vi "Conversie C2.vi"(0 "Array":string[](array[string])) -> (1 "12 bit LSB value (x)":i32, 2 "12 bit LSB value (y)":i32, 3 "12 bit LSB value (z)":i32, 4 "12 bit Field value (mT) X":dbl, 6 "12 bit Field value (mT) Y":dbl, 8 "12 bit Field value (mT) Z":dbl, 10 "12 bit temp (C)":dbl, 14 "12 bit LSB value (temp)":i32, 15 "FRM":i32)   [LabVIEW 2020]
panel:
  in  "Tab Control":enum32{"Page 1", "Page 2"}(tab)
  out "8 bit MSB value Z":i32
  out "8 bit Field value (mT) Z":dbl
  out "8 bit MSB value X":i32
  out "8 bit Field value (mT) X":dbl
  out "8 bit MSB value Y":i32
  out "8 bit Field value (mT) Y":dbl
  out "CH":i32
  out "T":i32
  out "FF":i32
  out "PD":i32
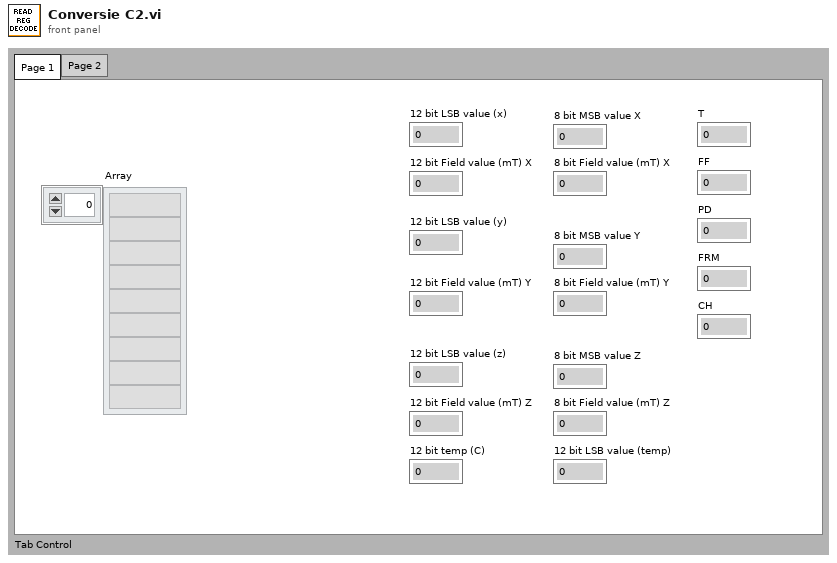
[diagram p1: front panel]
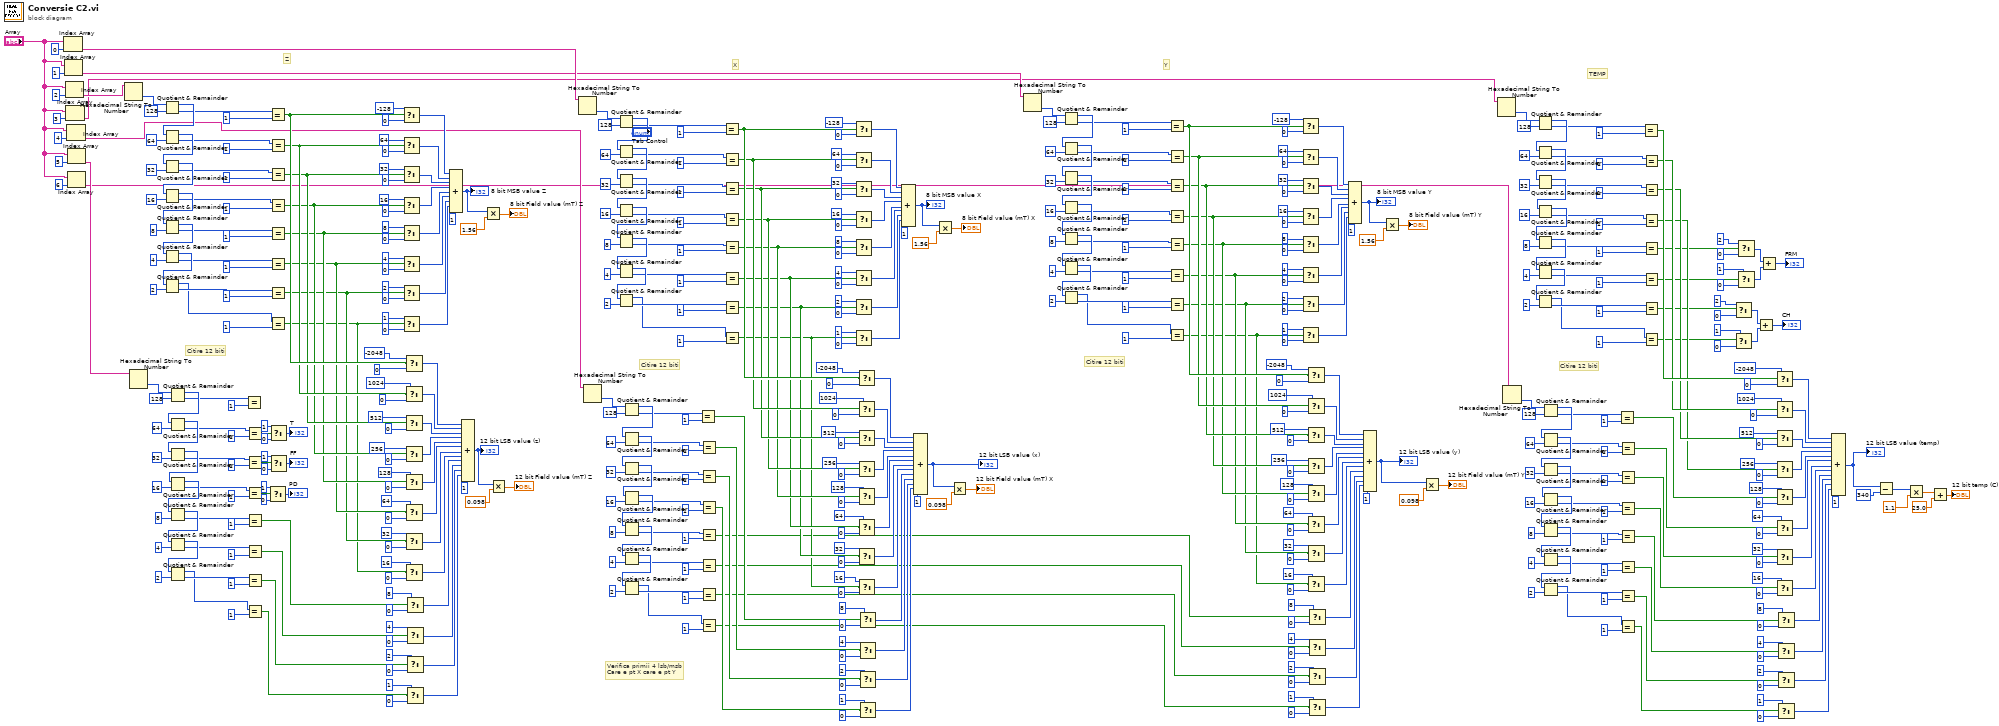
[diagram p0: block diagram]
diagram:
  # "Verifica primii 4 lsb/msb\nCare e pt X care e pt Y"
  # "TEMP"
  # "Y"
  # "X"
  # "Z"
  # "Citire 12 biti"
  # "Citire 12 biti"
  # "Citire 12 biti"
  # "Citire 12 biti"
  n1 = Index Array(array="Array", index=0) -> (element=w22:string)
  n2 = Index Array(array="Array", index=1) -> (element=w16:string)
  n3 = Index Array(array="Array", index=2) -> (element=w15:string)
  n4 = Index Array(array="Array", index=3) -> (element=w14:string)
  n5 = Index Array(array="Array", index=4) -> (element=w13:string)
  n6 = Index Array(array="Array", index=5) -> (element=w12:string)
  n7 = Index Array(array="Array", index=6) -> (element=w9:string)
  n8 = Hexadecimal String To Number(string=w15) -> (number=w522:u32)  [unwired: 2 in, 1 out]
  n9 = Hexadecimal String To Number(string=w12) -> (number=w466:u32)  [unwired: 2 in, 1 out]
  n10 = Quotient & Remainder(x=w522, y=u8 128) -> (x-y*floor(x/y)=w542:u32, floor(x/y)=w530:u32)
  n11 = Quotient & Remainder(x=w542, y=u8 64) -> (x-y*floor(x/y)=w541:u32, floor(x/y)=w524:u32)
  n12 = Quotient & Remainder(x=w541, y=u8 32) -> (x-y*floor(x/y)=w540:u32, floor(x/y)=w529:u32)
  n13 = Quotient & Remainder(x=w540, y=u8 16) -> (x-y*floor(x/y)=w539:u32, floor(x/y)=w528:u32)
  n14 = Quotient & Remainder(x=w539, y=u8 8) -> (x-y*floor(x/y)=w538:u32, floor(x/y)=w527:u32)
  n15 = Quotient & Remainder(x=w538, y=u8 4) -> (x-y*floor(x/y)=w537:u32, floor(x/y)=w526:u32)
  n16 = Quotient & Remainder(x=w537, y=u8 2) -> (x-y*floor(x/y)=w523:u32, floor(x/y)=w525:u32)
  n17 = Quotient & Remainder(x=w466, y=u8 128) -> (x-y*floor(x/y)=w486:u32, floor(x/y)=w474:u32)
  n18 = Quotient & Remainder(x=w486, y=u8 64) -> (x-y*floor(x/y)=w485:u32, floor(x/y)=w468:u32)
  n19 = Quotient & Remainder(x=w485, y=u8 32) -> (x-y*floor(x/y)=w484:u32, floor(x/y)=w473:u32)
  n20 = Quotient & Remainder(x=w484, y=u8 16) -> (x-y*floor(x/y)=w483:u32, floor(x/y)=w472:u32)
  n21 = Quotient & Remainder(x=w483, y=u8 8) -> (x-y*floor(x/y)=w482:u32, floor(x/y)=w471:u32)
  n22 = Quotient & Remainder(x=w482, y=u8 4) -> (x-y*floor(x/y)=w481:u32, floor(x/y)=w470:u32)
  n23 = Quotient & Remainder(x=w481, y=u8 2) -> (x-y*floor(x/y)=w467:u32, floor(x/y)=w469:u32)
  n24 = Equal?(x=w474, y=u8 1) -> ()  [unwired: 1 out]
  n25 = Equal?(x=w468, y=u8 1) -> (x = y?=w33:bool)
  n26 = Equal?(x=w473, y=u8 1) -> (x = y?=w28:bool)
  n27 = Equal?(x=w472, y=u8 1) -> (x = y?=w24:bool)
  n28 = Equal?(x=w471, y=u8 1) -> (x = y?=w156:bool)
  n29 = Equal?(x=w470, y=u8 1) -> (x = y?=w155:bool)
  n30 = Equal?(x=w469, y=u8 1) -> (x = y?=w154:bool)
  n31 = Equal?(x=w467, y=u8 1) -> (x = y?=w153:bool)
  n32 = Equal?(x=w530, y=u8 1) -> (x = y?=w164:bool)
  n33 = Select(t=u8 1 ("f"), s=w24, f=u8 0 ("t")) -> (s? t:f=→"PD":u8)
  n34 = Equal?(x=w524, y=u8 1) -> (x = y?=w163:bool)
  n35 = Equal?(x=w529, y=u8 1) -> (x = y?=w162:bool)
  n36 = Equal?(x=w528, y=u8 1) -> (x = y?=w161:bool)
  n37 = Equal?(x=w527, y=u8 1) -> (x = y?=w160:bool)
  n38 = Equal?(x=w526, y=u8 1) -> (x = y?=w159:bool)
  n39 = Equal?(x=w525, y=u8 1) -> (x = y?=w158:bool)
  n40 = Equal?(x=w523, y=u8 1) -> (x = y?=w157:bool)
  n41 = Select(t=u8 1 ("f"), s=w33, f=u8 0 ("t")) -> (s? t:f=→"T":u8)
  n42 = Select(t=u8 1 ("f"), s=w28, f=u8 0 ("t")) -> (s? t:f=→"FF":u8)
  n43 = Select(t=-128, s=w164, f=u8 0 ("t")) -> (s? t:f=w507:i32)
  n44 = Select(t=u8 64, s=w163, f=u8 0) -> (s? t:f=w506:u8)
  n45 = Select(t=u8 32, s=w162, f=u8 0) -> (s? t:f=w505:u8)
  n46 = Select(t=u8 16, s=w161, f=u8 0) -> (s? t:f=w504:u8)
  n47 = Select(t=u8 8, s=w160, f=u8 0) -> (s? t:f=w503:u8)
  n48 = Select(t=u8 4, s=w159, f=u8 0) -> (s? t:f=w502:u8)
  n49 = Select(t=u8 2, s=w158, f=u8 0) -> (s? t:f=w501:u8)
  n50 = Select(t=u8 1, s=w157, f=u8 0) -> (s? t:f=w500:u8)
  n51 = Select(t=-2048, s=w164, f=u8 0 ("t")) -> (s? t:f=w201:i32)
  n52 = Select(t=1024, s=w163, f=u8 0 ("t")) -> (s? t:f=w200:i32)
  n53 = Select(t=512, s=w162, f=u8 0 ("t")) -> (s? t:f=w199:i32)
  n54 = Select(t=256, s=w161, f=u8 0 ("t")) -> (s? t:f=w198:i32)
  n55 = Select(t=u8 128 ("f"), s=w160, f=u8 0 ("t")) -> (s? t:f=w197:u8)
  n56 = Select(t=u8 64 ("f"), s=w159, f=u8 0 ("t")) -> (s? t:f=w196:u8)
  n57 = Select(t=u8 32 ("f"), s=w158, f=u8 0 ("t")) -> (s? t:f=w195:u8)
  n58 = Select(t=u8 16 ("f"), s=w157, f=u8 0 ("t")) -> (s? t:f=w194:u8)
  n59 = Select(t=u8 8 ("f"), s=w156, f=u8 0 ("t")) -> (s? t:f=w192:u8)
  n60 = Select(t=u8 4 ("f"), s=w155, f=u8 0 ("t")) -> (s? t:f=w191:u8)
  n61 = Select(t=u8 2 ("f"), s=w154, f=u8 0 ("t")) -> (s? t:f=w190:u8)
  n62 = Select(t=u8 1 ("f"), s=w153, f=u8 0 ("t")) -> (s? t:f=w189:u8)
  n63 = Compound Arithmetic op=ADD(w507, w506, w505, w504, w503, w502, w501, w500, u8 1 ("Input")) -> (w498:i32)
  "8 bit MSB value Z" <- w498
  n64 = Compound Arithmetic op=ADD(w201, w200, w199, w198, w197, w196, w195, w194, w192, w191, w190, w189, u8 1 ("Input")) -> (w152:i32)
  "12 bit LSB value (z)" <- w152
  n65 = Multiply(x=w498, y=1.56) -> (x*y=→"8 bit Field value (mT) Z":dbl)
  n66 = Multiply(x=w152, y=0.098) -> (x*y=→"12 bit Field value (mT) Z":dbl)
  n67 = Hexadecimal String To Number(string=w22) -> (number=w434:u32)  [unwired: 2 in, 1 out]
  n68 = Hexadecimal String To Number(string=w13) -> (number=w378:u32)  [unwired: 2 in, 1 out]
  n69 = Quotient & Remainder(x=w434, y=u8 128) -> (x-y*floor(x/y)=w454:u32, floor(x/y)=w442:u32)
  n70 = Quotient & Remainder(x=w454, y=u8 64) -> (x-y*floor(x/y)=w453:u32, floor(x/y)=w436:u32)
  n71 = Quotient & Remainder(x=w453, y=u8 32) -> (x-y*floor(x/y)=w452:u32, floor(x/y)=w441:u32)
  n72 = Quotient & Remainder(x=w452, y=u8 16) -> (x-y*floor(x/y)=w451:u32, floor(x/y)=w440:u32)
  n73 = Quotient & Remainder(x=w451, y=u8 8) -> (x-y*floor(x/y)=w450:u32, floor(x/y)=w439:u32)
  n74 = Quotient & Remainder(x=w450, y=u8 4) -> (x-y*floor(x/y)=w449:u32, floor(x/y)=w438:u32)
  n75 = Quotient & Remainder(x=w449, y=u8 2) -> (x-y*floor(x/y)=w435:u32, floor(x/y)=w437:u32)
  n76 = Quotient & Remainder(x=w378, y=u8 128) -> (x-y*floor(x/y)=w398:u32, floor(x/y)=w386:u32)
  n77 = Quotient & Remainder(x=w398, y=u8 64) -> (x-y*floor(x/y)=w397:u32, floor(x/y)=w380:u32)
  n78 = Quotient & Remainder(x=w397, y=u8 32) -> (x-y*floor(x/y)=w396:u32, floor(x/y)=w385:u32)
  n79 = Quotient & Remainder(x=w396, y=u8 16) -> (x-y*floor(x/y)=w395:u32, floor(x/y)=w384:u32)
  n80 = Quotient & Remainder(x=w395, y=u8 8) -> (x-y*floor(x/y)=w394:u32, floor(x/y)=w383:u32)
  n81 = Quotient & Remainder(x=w394, y=u8 4) -> (x-y*floor(x/y)=w393:u32, floor(x/y)=w382:u32)
  n82 = Quotient & Remainder(x=w393, y=u8 2) -> (x-y*floor(x/y)=w379:u32, floor(x/y)=w381:u32)
  n83 = Equal?(x=w386, y=u8 1) -> (x = y?=w8:bool)
  n84 = Equal?(x=w380, y=u8 1) -> (x = y?=w7:bool)
  n85 = Equal?(x=w385, y=u8 1) -> (x = y?=w6:bool)
  n86 = Equal?(x=w384, y=u8 1) -> (x = y?=w5:bool)
  n87 = Equal?(x=w383, y=u8 1) -> (x = y?=w4:bool)
  n88 = Equal?(x=w382, y=u8 1) -> (x = y?=w3:bool)
  n89 = Equal?(x=w381, y=u8 1) -> (x = y?=w2:bool)
  n90 = Equal?(x=w379, y=u8 1) -> (x = y?=w1:bool)
  n91 = Equal?(x=w442, y=u8 1) -> (x = y?=w115:bool)
  n92 = Equal?(x=w436, y=u8 1) -> (x = y?=w114:bool)
  n93 = Equal?(x=w441, y=u8 1) -> (x = y?=w113:bool)
  n94 = Equal?(x=w440, y=u8 1) -> (x = y?=w112:bool)
  n95 = Equal?(x=w439, y=u8 1) -> (x = y?=w111:bool)
  n96 = Equal?(x=w438, y=u8 1) -> (x = y?=w110:bool)
  n97 = Equal?(x=w437, y=u8 1) -> (x = y?=w109:bool)
  n98 = Equal?(x=w435, y=u8 1) -> (x = y?=w108:bool)
  n99 = Select(t=-128, s=w115, f=u8 0 ("t")) -> (s? t:f=w419:i32)
  n100 = Select(t=u8 64, s=w114, f=u8 0) -> (s? t:f=w418:u8)
  n101 = Select(t=u8 32, s=w113, f=u8 0) -> (s? t:f=w417:u8)
  n102 = Select(t=u8 16, s=w112, f=u8 0) -> (s? t:f=w416:u8)
  n103 = Select(t=u8 8, s=w111, f=u8 0) -> (s? t:f=w415:u8)
  n104 = Select(t=u8 4, s=w110, f=u8 0) -> (s? t:f=w414:u8)
  n105 = Select(t=u8 2, s=w109, f=u8 0) -> (s? t:f=w413:u8)
  n106 = Select(t=u8 1, s=w108, f=u8 0) -> (s? t:f=w412:u8)
  n107 = Select(t=-2048, s=w115, f=u8 0 ("t")) -> (s? t:f=w151:i32)
  n108 = Select(t=1024, s=w114, f=u8 0 ("t")) -> (s? t:f=w150:i32)
  n109 = Select(t=512, s=w113, f=u8 0 ("t")) -> (s? t:f=w149:i32)
  n110 = Select(t=256, s=w112, f=u8 0 ("t")) -> (s? t:f=w148:i32)
  n111 = Select(t=u8 128 ("f"), s=w111, f=u8 0 ("t")) -> (s? t:f=w147:u8)
  n112 = Select(t=u8 64 ("f"), s=w110, f=u8 0 ("t")) -> (s? t:f=w146:u8)
  n113 = Select(t=u8 32 ("f"), s=w109, f=u8 0 ("t")) -> (s? t:f=w145:u8)
  n114 = Select(t=u8 16 ("f"), s=w108, f=u8 0 ("t")) -> (s? t:f=w144:u8)
  n115 = Select(t=u8 8 ("f"), s=w8, f=u8 0 ("t")) -> (s? t:f=w142:u8)
  n116 = Select(t=u8 4 ("f"), s=w7, f=u8 0 ("t")) -> (s? t:f=w141:u8)
  n117 = Select(t=u8 2 ("f"), s=w6, f=u8 0 ("t")) -> (s? t:f=w140:u8)
  n118 = Select(t=u8 1 ("f"), s=w5, f=u8 0 ("t")) -> (s? t:f=w139:u8)
  n119 = Compound Arithmetic op=ADD(w419, w418, w417, w416, w415, w414, w413, w412, u8 1 ("Input")) -> (w410:i32)
  "8 bit MSB value X" <- w410
  n120 = Compound Arithmetic op=ADD(w151, w150, w149, w148, w147, w146, w145, w144, w142, w141, w140, w139, u8 1 ("Input")) -> (w107:i32)
  "12 bit LSB value (x)" <- w107
  n121 = Multiply(x=w410, y=1.56) -> (x*y=→"8 bit Field value (mT) X":dbl)
  n122 = Multiply(x=w107, y=0.098) -> (x*y=→"12 bit Field value (mT) X":dbl)
  n123 = Hexadecimal String To Number(string=w16) -> (number=w346:u32)  [unwired: 2 in, 1 out]
  n124 = Quotient & Remainder(x=w346, y=u8 128) -> (x-y*floor(x/y)=w366:u32, floor(x/y)=w354:u32)
  n125 = Quotient & Remainder(x=w366, y=u8 64) -> (x-y*floor(x/y)=w365:u32, floor(x/y)=w348:u32)
  n126 = Quotient & Remainder(x=w365, y=u8 32) -> (x-y*floor(x/y)=w364:u32, floor(x/y)=w353:u32)
  n127 = Quotient & Remainder(x=w364, y=u8 16) -> (x-y*floor(x/y)=w363:u32, floor(x/y)=w352:u32)
  n128 = Quotient & Remainder(x=w363, y=u8 8) -> (x-y*floor(x/y)=w362:u32, floor(x/y)=w351:u32)
  n129 = Quotient & Remainder(x=w362, y=u8 4) -> (x-y*floor(x/y)=w361:u32, floor(x/y)=w350:u32)
  n130 = Quotient & Remainder(x=w361, y=u8 2) -> (x-y*floor(x/y)=w347:u32, floor(x/y)=w349:u32)
  n131 = Equal?(x=w354, y=u8 1) -> (x = y?=w70:bool)
  n132 = Equal?(x=w348, y=u8 1) -> (x = y?=w69:bool)
  n133 = Equal?(x=w353, y=u8 1) -> (x = y?=w68:bool)
  n134 = Equal?(x=w352, y=u8 1) -> (x = y?=w67:bool)
  n135 = Equal?(x=w351, y=u8 1) -> (x = y?=w66:bool)
  n136 = Equal?(x=w350, y=u8 1) -> (x = y?=w65:bool)
  n137 = Equal?(x=w349, y=u8 1) -> (x = y?=w64:bool)
  n138 = Equal?(x=w347, y=u8 1) -> (x = y?=w63:bool)
  n139 = Select(t=-128, s=w70, f=u8 0 ("t")) -> (s? t:f=w331:i32)
  n140 = Select(t=u8 64, s=w69, f=u8 0) -> (s? t:f=w330:u8)
  n141 = Select(t=u8 32, s=w68, f=u8 0) -> (s? t:f=w329:u8)
  n142 = Select(t=u8 16, s=w67, f=u8 0) -> (s? t:f=w328:u8)
  n143 = Select(t=u8 8, s=w66, f=u8 0) -> (s? t:f=w327:u8)
  n144 = Select(t=u8 4, s=w65, f=u8 0) -> (s? t:f=w326:u8)
  n145 = Select(t=u8 2, s=w64, f=u8 0) -> (s? t:f=w325:u8)
  n146 = Select(t=u8 1, s=w63, f=u8 0) -> (s? t:f=w324:u8)
  n147 = Select(t=-2048, s=w70, f=u8 0 ("t")) -> (s? t:f=w106:i32)
  n148 = Select(t=1024, s=w69, f=u8 0 ("t")) -> (s? t:f=w105:i32)
  n149 = Select(t=512, s=w68, f=u8 0 ("t")) -> (s? t:f=w104:i32)
  n150 = Select(t=256, s=w67, f=u8 0 ("t")) -> (s? t:f=w103:i32)
  n151 = Select(t=u8 128 ("f"), s=w66, f=u8 0 ("t")) -> (s? t:f=w102:u8)
  n152 = Select(t=u8 64 ("f"), s=w65, f=u8 0 ("t")) -> (s? t:f=w101:u8)
  n153 = Select(t=u8 32 ("f"), s=w64, f=u8 0 ("t")) -> (s? t:f=w100:u8)
  n154 = Select(t=u8 16 ("f"), s=w63, f=u8 0 ("t")) -> (s? t:f=w99:u8)
  n155 = Select(t=u8 8 ("f"), s=w4, f=u8 0 ("t")) -> (s? t:f=w97:u8)
  n156 = Select(t=u8 4 ("f"), s=w3, f=u8 0 ("t")) -> (s? t:f=w96:u8)
  n157 = Select(t=u8 2 ("f"), s=w2, f=u8 0 ("t")) -> (s? t:f=w95:u8)
  n158 = Select(t=u8 1 ("f"), s=w1, f=u8 0 ("t")) -> (s? t:f=w94:u8)
  n159 = Compound Arithmetic op=ADD(w331, w330, w329, w328, w327, w326, w325, w324, u8 1 ("Input")) -> (w322:i32)
  "8 bit MSB value Y" <- w322
  n160 = Compound Arithmetic op=ADD(w106, w105, w104, w103, w102, w101, w100, w99, w97, w96, w95, w94, u8 1 ("Input")) -> (w62:i32)
  "12 bit LSB value (y)" <- w62
  n161 = Multiply(x=w322, y=1.56) -> (x*y=→"8 bit Field value (mT) Y":dbl)
  n162 = Multiply(x=w62, y=0.098) -> (x*y=→"12 bit Field value (mT) Y":dbl)
  n163 = Hexadecimal String To Number(string=w14) -> (number=w288:u32)  [unwired: 2 in, 1 out]
  n164 = Hexadecimal String To Number(string=w9) -> (number=w258:u32)  [unwired: 2 in, 1 out]
  n165 = Quotient & Remainder(x=w288, y=u8 128) -> (x-y*floor(x/y)=w308:u32, floor(x/y)=w296:u32)
  n166 = Quotient & Remainder(x=w308, y=u8 64) -> (x-y*floor(x/y)=w307:u32, floor(x/y)=w290:u32)
  n167 = Quotient & Remainder(x=w307, y=u8 32) -> (x-y*floor(x/y)=w306:u32, floor(x/y)=w295:u32)
  n168 = Quotient & Remainder(x=w306, y=u8 16) -> (x-y*floor(x/y)=w305:u32, floor(x/y)=w294:u32)
  n169 = Quotient & Remainder(x=w305, y=u8 8) -> (x-y*floor(x/y)=w304:u32, floor(x/y)=w293:u32)
  n170 = Quotient & Remainder(x=w304, y=u8 4) -> (x-y*floor(x/y)=w303:u32, floor(x/y)=w292:u32)
  n171 = Quotient & Remainder(x=w303, y=u8 2) -> (x-y*floor(x/y)=w289:u32, floor(x/y)=w291:u32)
  n172 = Quotient & Remainder(x=w258, y=u8 128) -> (x-y*floor(x/y)=w278:u32, floor(x/y)=w266:u32)
  n173 = Quotient & Remainder(x=w278, y=u8 64) -> (x-y*floor(x/y)=w277:u32, floor(x/y)=w260:u32)
  n174 = Quotient & Remainder(x=w277, y=u8 32) -> (x-y*floor(x/y)=w276:u32, floor(x/y)=w265:u32)
  n175 = Quotient & Remainder(x=w276, y=u8 16) -> (x-y*floor(x/y)=w275:u32, floor(x/y)=w264:u32)
  n176 = Quotient & Remainder(x=w275, y=u8 8) -> (x-y*floor(x/y)=w274:u32, floor(x/y)=w263:u32)
  n177 = Quotient & Remainder(x=w274, y=u8 4) -> (x-y*floor(x/y)=w273:u32, floor(x/y)=w262:u32)
  n178 = Quotient & Remainder(x=w273, y=u8 2) -> (x-y*floor(x/y)=w259:u32, floor(x/y)=w261:u32)
  n179 = Equal?(x=w266, y=u8 1) -> (x = y?=w235:bool)
  n180 = Equal?(x=w260, y=u8 1) -> (x = y?=w234:bool)
  n181 = Equal?(x=w265, y=u8 1) -> (x = y?=w233:bool)
  n182 = Equal?(x=w264, y=u8 1) -> (x = y?=w232:bool)
  n183 = Equal?(x=w263, y=u8 1) -> (x = y?=w254:bool)
  n184 = Equal?(x=w262, y=u8 1) -> (x = y?=w255:bool)
  n185 = Equal?(x=w261, y=u8 1) -> (x = y?=w256:bool)
  n186 = Equal?(x=w259, y=u8 1) -> (x = y?=w257:bool)
  n187 = Equal?(x=w296, y=u8 1) -> (x = y?=w245:bool)
  n188 = Equal?(x=w290, y=u8 1) -> (x = y?=w244:bool)
  n189 = Equal?(x=w295, y=u8 1) -> (x = y?=w243:bool)
  n190 = Equal?(x=w294, y=u8 1) -> (x = y?=w242:bool)
  n191 = Equal?(x=w293, y=u8 1) -> (x = y?=w49:bool)
  n192 = Equal?(x=w292, y=u8 1) -> (x = y?=w48:bool)
  n193 = Equal?(x=w291, y=u8 1) -> (x = y?=w37:bool)
  n194 = Equal?(x=w289, y=u8 1) -> (x = y?=w36:bool)
  n195 = Select(t=u8 2 ("f"), s=w37, f=u8 0 ("t")) -> (s? t:f=w39:u8)
  n196 = Select(t=u8 1 ("f"), s=w36, f=u8 0 ("t")) -> (s? t:f=w40:u8)
  n197 = Select(t=u8 2 ("f"), s=w49, f=u8 0 ("t")) -> (s? t:f=w46:u8)
  n198 = Select(t=u8 1 ("f"), s=w48, f=u8 0 ("t")) -> (s? t:f=w47:u8)
  n199 = Add(x=w39, y=w40) -> (x+y=→"CH":u8)
  n200 = Add(x=w46, y=w47) -> (x+y=→"FRM":u8)
  n201 = Select(t=-2048, s=w245, f=u8 0 ("t")) -> (s? t:f=w253:i32)
  n202 = Select(t=1024, s=w244, f=u8 0 ("t")) -> (s? t:f=w252:i32)
  n203 = Select(t=512, s=w243, f=u8 0 ("t")) -> (s? t:f=w251:i32)
  n204 = Select(t=256, s=w242, f=u8 0 ("t")) -> (s? t:f=w250:i32)
  n205 = Select(t=u8 128 ("f"), s=w235, f=u8 0 ("t")) -> (s? t:f=w249:u8)
  n206 = Select(t=u8 64 ("f"), s=w234, f=u8 0 ("t")) -> (s? t:f=w248:u8)
  n207 = Select(t=u8 32 ("f"), s=w233, f=u8 0 ("t")) -> (s? t:f=w247:u8)
  n208 = Select(t=u8 16 ("f"), s=w232, f=u8 0 ("t")) -> (s? t:f=w246:u8)
  n209 = Select(t=u8 8 ("f"), s=w254, f=u8 0 ("t")) -> (s? t:f=w240:u8)
  n210 = Select(t=u8 4 ("f"), s=w255, f=u8 0 ("t")) -> (s? t:f=w239:u8)
  n211 = Select(t=u8 2 ("f"), s=w256, f=u8 0 ("t")) -> (s? t:f=w238:u8)
  n212 = Select(t=u8 1 ("f"), s=w257, f=u8 0 ("t")) -> (s? t:f=w237:u8)
  n213 = Compound Arithmetic op=ADD(w253, w252, w251, w250, w249, w248, w247, w246, w240, w239, w238, w237, u8 1 ("Input")) -> (w231:i32)
  "12 bit LSB value (temp)" <- w231
  n214 = Subtract(x=w231, y=340) -> (x-y=w229:i32)
  n215 = Multiply(x=w229, y=1.1) -> (x*y=w228:dbl)
  n216 = Add(x=w228, y=25.0) -> (x+y=→"12 bit temp (C)":dbl)
